vi "Power Supply Manual Ctl Programming.vi"() -> ()   [LabVIEW 2022 SP3]
uses:
  HMP4000 Communication/HMP4040_ChannelControl.ctl
  <vilib>/DAQmx/write.llb/DAQmx Write (Digital Bool 1Line 1Point).vi
  <vilib>/DAQmx/miscellaneous.llb/DAQmx Fill In Error Info.vi
panel:
  in  "error in (no error)":errorcluster
  in  "Control Power":bool
  in  "Programming Pin":bool
  out "CH2 Voltage":dbl(knob) caption="Voltage Value" scale=0.0..30.0
  out "CH2 Current":dbl(knob) caption="Current" scale=0.0..3.0
  in  "stop":bool
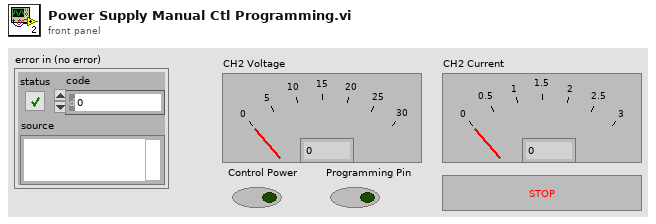
[diagram p1: front panel]
types:
  T1 = typedef "HMP4040_ChannelControl.ctl" = cluster{"CH1 Voltage":dbl, "CH1 Current":dbl, "CH1 Output":bool, "CH2 Voltage":dbl, "CH2 Current":dbl, "CH2 Output":bool, "CH3 Voltage":dbl, "CH3 Current":dbl, "CH3 Output":bool, "CH4 Voltage":dbl, "CH4 Current":dbl, "CH4 Output":bool, "Master Output":bool}
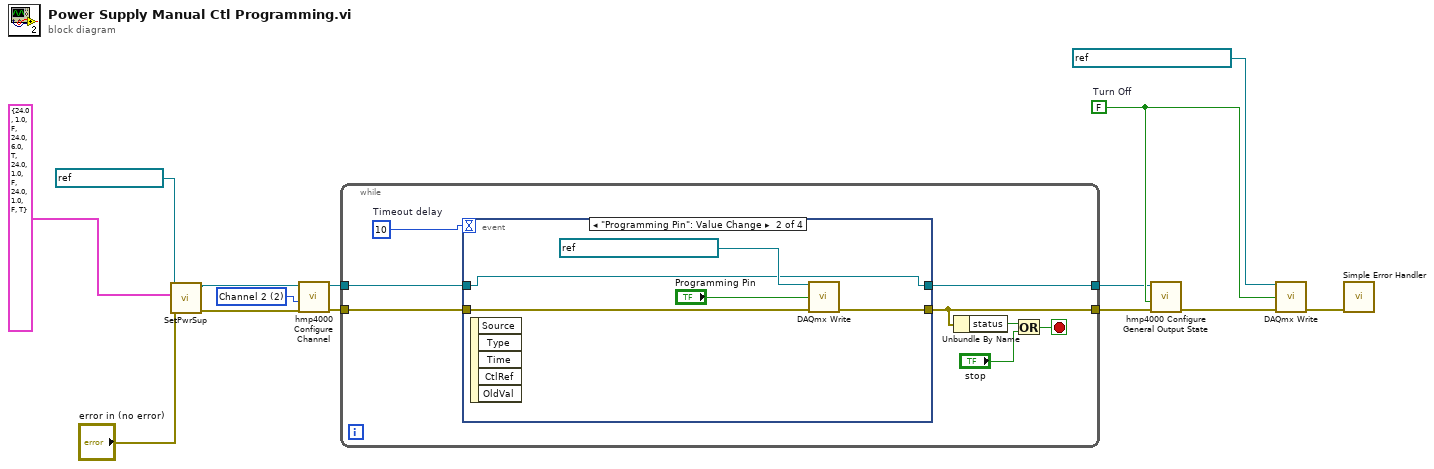
[diagram p0: block diagram]
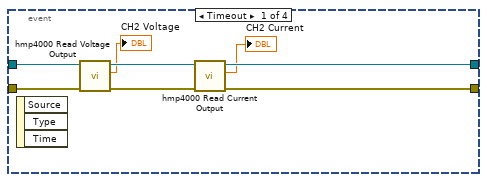
[diagram p2: hidden frame]
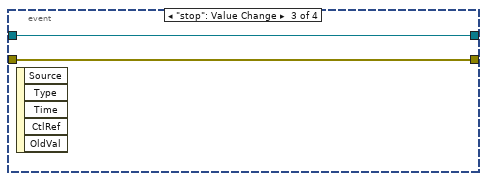
[diagram p3: hidden frame]
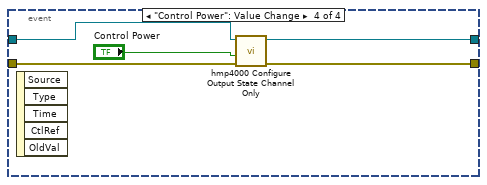
[diagram p4: hidden frame]
diagram:
  w8 = 2 items=["Channel 1"=1, "Channel 2"=2, "Channel 3"=3, "Channel 4"=4] ("Channel (Channel 1)")
  w10 = FALSE  # Turn Off
  n1 = call "SetPwrSup.vi"("error in (no error)"="error in (no error)", "HMP4040 Channel Settings"=T1 {"CH1 Voltage"=24.0, "CH1 Current"=1.0, "CH1 Output"=FALSE, "CH2 Voltage"=24.0, "CH2 Current"=6.0, "CH2 Output"=TRUE, "CH3 Voltage"=24.0, "CH3 Current"=1.0, "CH3 Output"=FALSE, "CH4 Voltage"=24.0, "CH4 Current"=1.0, "CH4 Output"=FALSE, "Master Output"=TRUE}, "HMP4040 IN"=refnum<visa-resource-name> "HMP4040_FTS2") -> ("error out"=w5:errorcluster, "HMP4040_OUT"=w1:refnum<visa-resource-name>)  [unwired: 7 in]
  n2 = call <instrlib>:"hmp4000 Configure Channel.vi"("error in (no error)"=w5, "Channel (Channel 1)"=w8, "VISA resource name"=w1) -> ("error out"=w6:errorcluster, "VISA resource name out"=w7:refnum<visa-resource-name>)  [unwired: 7 in]
  n3 = while {
    tunnel: w6 -> [w18]
    tunnel: w7 -> [w22]
    tunnel: [w16] -> w9
    tunnel: [w20] -> w11
    stop <- w21 stop-if-true
    w19 = 10  # Timeout delay
    n4 = event shown="[1] \"Programming Pin\": Value Change" {
      selector: _ -> [_ _ _ _]
      dyn-events: _ -> [_ _ _ _]
      timeout: w19 -> [_ _ _ _]
      tunnel: [w25 w31 w36 w41] -> w16
      tunnel: w18 -> [w29 w32 w37 w38]
      tunnel: w22 -> [w30 w31 w36 w39]
      tunnel: [w26 w34 w37 w42] -> w20
      event Timeout {
        n5 = event-data() -> ()  [unwired: 1 in, 3 out]
        n6 = call <instrlib>:"hmp4000 Read Voltage Output.vi"("error in (no error)"=w29, "VISA resource name"=w30) -> ("error out"=w27:errorcluster, "Voltage Value"=→"CH2 Voltage":dbl, "VISA resource name out"=w28:refnum<visa-resource-name>)  [unwired: 7 in]
        n7 = call <instrlib>:"hmp4000 Read Current Output.vi"("error in (no error)"=w27, "VISA resource name"=w28) -> ("error out"=w26:errorcluster, "Current Value"=→"CH2 Current":dbl, "VISA resource name out"=w25:refnum<visa-resource-name>)  [unwired: 7 in]
      }
      event "Programming Pin": Value Change {
        n8 = event-data() -> ()  [unwired: 1 in, 5 out]
        n9 = call-poly <vilib>:"DAQmx Write.vi"("task/channels in"=refnum<k21> "FTS2_ProgrammingRelay", "data"="Programming Pin", "error in"=w32) -> ("error out"=w34:errorcluster)  [unwired: 10 in, 2 out]
      }
      event "stop": Value Change {
        n10 = event-data() -> ()  [unwired: 1 in, 5 out]
      }
      event "Control Power": Value Change {
        n11 = event-data() -> ()  [unwired: 1 in, 5 out]
        n12 = call <instrlib>:"hmp4000 Configure Output State Channel Only.vi"("error in (no error)"=w38, "Output State (Off)"="Control Power", "VISA resource name"=w39) -> ("error out"=w42:errorcluster, "VISA resource name out"=w41:refnum<visa-resource-name>)  [unwired: 7 in]
      }
    }
    n13 = Unbundle By Name(w20) -> ("status"=w17:bool)
    n14 = Or(x=w17, y="stop") -> (x .or. y?=w21:bool)
  }
  n15 = call <instrlib>:"hmp4000 Configure General Output State.vi"("error in (no error)"=w11, "Output State (Off)"=w10, "VISA resource name"=w9) -> ("error out"=w12:errorcluster)  [unwired: 7 in, 1 out]
  n16 = call-poly <vilib>:"DAQmx Write.vi"("task/channels in"=refnum<k21> "FTS2_ProgrammingRelay", "data"=w10, "error in"=w12) -> ("error out"=w13:errorcluster)  [unwired: 10 in, 2 out]
  n17 = call <vilib>:"Simple Error Handler.vi"("error in (no error)"=w13) -> ()  [unwired: 4 in, 5 out]
